vi "Discover Unique Names of Dependencies.vi"(0 "NI Build Specification_LV In":refnum<class "NI Build Specification_LV.lvclass">) -> (4 "NI Build Specification_LV Out":refnum<class "NI Build Specification_LV.lvclass">)   [LabVIEW 2017, in "CL_G3_VIComponentBuilder.lvlib" / "NI Build Specification_LV.lvclass"]
doc: "Interrogates this export's dependencies for thier unique names (as opposed to the product name of the dependency). The unique names are used when assembling the working set of exports in order to prevent name collisions and allow the build analyzer to determine the build order."
uses:
  NI Build Specification_LV.lvclass
  Exports/Export.lvclass
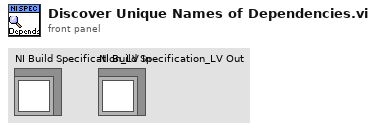
[diagram p1: front panel]
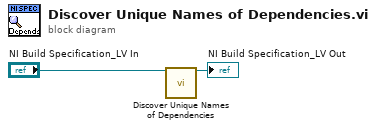
[diagram p0: block diagram]
diagram:
  n1 = call-parent "Discover Unique Names of Dependencies.vi"("Export In"="NI Build Specification_LV In") -> ("Export Out"=→"NI Build Specification_LV Out":refnum<class "NI Build Specification_LV.lvclass">)  [unwired: 14 in]
